vi "Single Channel FPGA with C.vi"(5 "Reset":bool, 6 "DIR":bool, 7 "Period (Ticks)":u32=4000, 8 "STBY":bool, 9 "ENA":bool, 10 "Duty":fxp<+,32,0>, 11 "IO Channels":T2={"PWM In"="", "Direction"="", "ENA"="", "Encoder C"="", "Encoder B"="Connector1/DIO20", "Encoder A"="", "STBY"=""}) -> (2 "JumpBy2Error":i16, 3 "Position":i32)   [LabVIEW 2018]
uses:
  <vilib>/eio/EIONode/EIONode.xnode
  jmslib.lvlib
  kevLib2010.lvlib
  Control 1.ctl
  <vilib>/rvi/eio/common/nirviEmuTemplateMethod_errors.vi
panel:
  out "I/O Item":bool
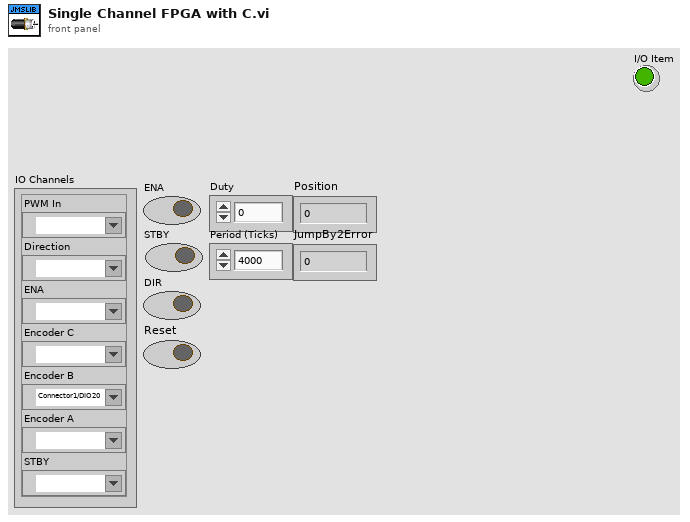
[diagram p1: front panel]
types:
  T1 = typedef "Control 1.ctl" = refnum<k21>
  T2 = cluster{"PWM In":refnum<k21>, "Direction":refnum<k21>, "ENA":refnum<k21>, "Encoder C":T1, "Encoder B":refnum<k21>, "Encoder A":refnum<k21>, "STBY":refnum<k21>}
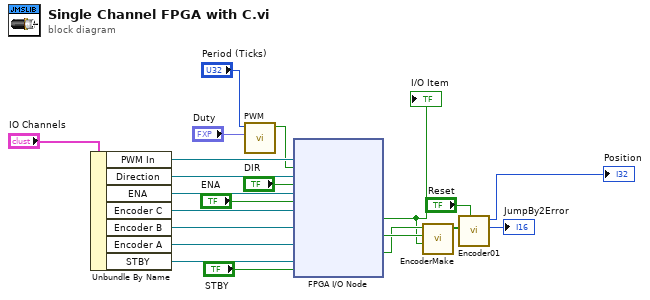
[diagram p0: block diagram]
diagram:
  n1 = Unbundle By Name("IO Channels") -> ("PWM In"=w12:refnum<k21>, "Direction"=w11:refnum<k21>, "ENA"=w10:refnum<k21>, "Encoder C"=w8:T1, "Encoder B"=w7:refnum<k21>, "Encoder A"=w6:refnum<k21>, "STBY"=w5:refnum<k21>)
  n2 = call "PWM.vi"("Duty Cycle"="Duty", "Period (Ticks)"="Period (Ticks)") -> ("PWM Out"=w9:bool)  [unwired: 8 in, 1 out]
  n3 = xnode "FPGA I/O Node"("I/O Item"=w9, "FPGA I/O In"=w12, "I/O Item"="DIR", "FPGA I/O In"=w11, "I/O Item"="ENA", "FPGA I/O In"=w10, "FPGA I/O In"=w8, "FPGA I/O In"=w7, "FPGA I/O In"=w6, "I/O Item"="STBY", "FPGA I/O In"=w5) -> ("I/O Item"=w1:bool, "I/O Item"=w18:bool, "I/O Item"=w17:bool)  [unwired: 7 out]
  "I/O Item" <- w1
  n4 = call "EncoderMake.vi"("C"=w1, "B"=w18, "A"=w17) -> ("Encoder Array"=w16:bool[])  [unwired: 8 in]
  n5 = call "Encoder01.vi"("ForceReset"="Reset", "Encoder Array"=w16) -> ("JumpBy2Error"=→"JumpBy2Error":i16, "Position"=→"Position":i32)  [unwired: 6 in, 2 out]
